vi "TRITON_PID_COMMAND.vi"(1 "D":dbl, 2 "I":dbl, 3 "P":dbl, 4 "Control Channel":i32) -> (0 "PID Command":string)   [LabVIEW 2009]
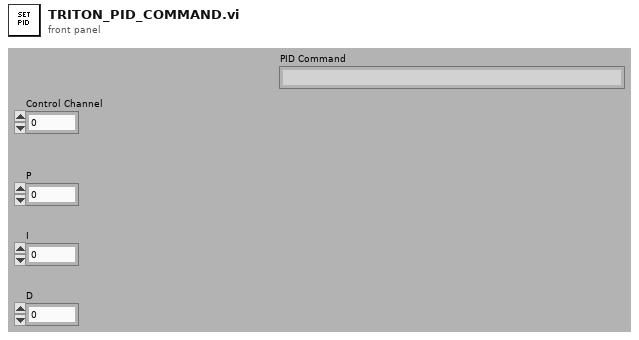
[diagram p1: front panel]
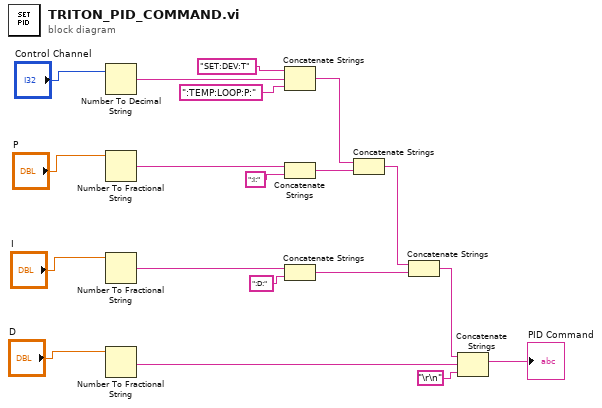
[diagram p0: block diagram]
diagram:
  n1 = Number To Decimal String(number="Control Channel") -> (decimal integer string=w14:string)  [unwired: 1 in]
  n2 = Number To Fractional String(number="P") -> (F-format string=w12:string)  [unwired: 3 in]
  n3 = Number To Fractional String(number="I") -> (F-format string=w10:string)  [unwired: 3 in]
  n4 = Number To Fractional String(number="D") -> (F-format string=w3:string)  [unwired: 3 in]
  n5 = Concatenate Strings("SET:DEV:T", w14, ":TEMP:LOOP:P:") -> (w8:string)
  n6 = Concatenate Strings(w12, ":I:") -> (w7:string)
  n7 = Concatenate Strings(w10, ":D:") -> (w5:string)
  n8 = Concatenate Strings(w8, w7) -> (w6:string)
  n9 = Concatenate Strings(w6, w5) -> (w4:string)
  n10 = Concatenate Strings(w4, w3, "\r\n") -> (→"PID Command":string)
